vi "Laser Rough Cutting.vi"(0 "configuration file path":path caption="配置文件的路径", 1 "rough cutting msic":T1) -> ()   [LabVIEW 2014]
uses:
  Ctl.xio/rough cutting msic ctl.ctl
  SubVIS.xio/DataSocket/DataSocket_Tags.ctl
  Ctl.xio/part type.ctl
  SubVIS.xio/Creat Write List VI's/DefCtrl/Station.ctl
  SubVIS.xio/DataSocket/Write PLC Vars/Write String Var in.vi
  <vilib>/Utility/file.llb/Read From Spreadsheet File (string).vi
  SubVIS.xio/DataSocket/Write PLC Vars/Write Bool Var in.vi
  SubVIS.xio/DataSocket/Read PLC Vars/Read String Var.vi
  SubVIS.xio/DataSocket/Write PLC Vars/Write Dbl Var in.vi
  SubVIS.xio/DataSocket/Read PLC Vars/Read Bool Var.vi
  SubVIS.xio/DataSocket/Read PLC Vars/Read U32 Var.vi
panel:
  in  "SQL information":string
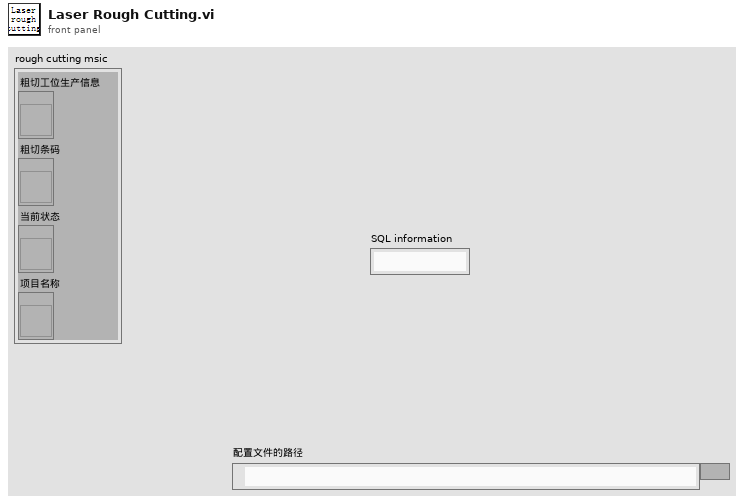
[diagram p1: front panel]
types:
  T1 = cluster{"粗切工位生产信息":refnum<vi>, "粗切条码":refnum<vi>, "当前状态":refnum<vi>, "项目名称":refnum<vi>}
  T2 = typedef "Station.ctl" = enum16{"粗切工位", "热处理工位", "精切工位", "PDF焊接工位", "打凹点预载力工位", "收卷工位", "EOL工位"}
  T3 = typedef "rough cutting msic ctl.ctl" = cluster{"configuration file path":path, "DsOut":T4[], "scanner coms or ip":string, "BarCode":string, "scanner resource name out":refnum<visa-resource-name>, "Hopper car information":cluster{"Hopper car code":string, "Hopper car No":string, "plate No":string}, "pallet.produced number":i32, "SQL information":string, "Database":string[], "Serial number":i32, "database path":path, "rough cutting msic":cluster{"粗切工位生产信息":refnum<vi>, "粗切条码":refnum<vi>, "当前状态":refnum<vi>, "项目名称":refnum<vi>}, "part type":T5, "scanner ip ID":refnum<k5>, "Number of scans ":u8}
  T4 = typedef "DataSocket_Tags.ctl" = cluster{"Ds ID":refnum<k13>, "Tag":string}
  T5 = typedef "part type.ctl" = cluster{"项目号":string, "物料代码":string, "零件号":string, "供应商编码":string, "产线编码":string, "客户代码":string, "颜色代码":string, "托盘上限":i32, "加热温度":string, "加热时长":string, "EOL Stations":string}
  T6 = cluster{"Hopper car code":string, "Hopper car No":string, "plate No":string}
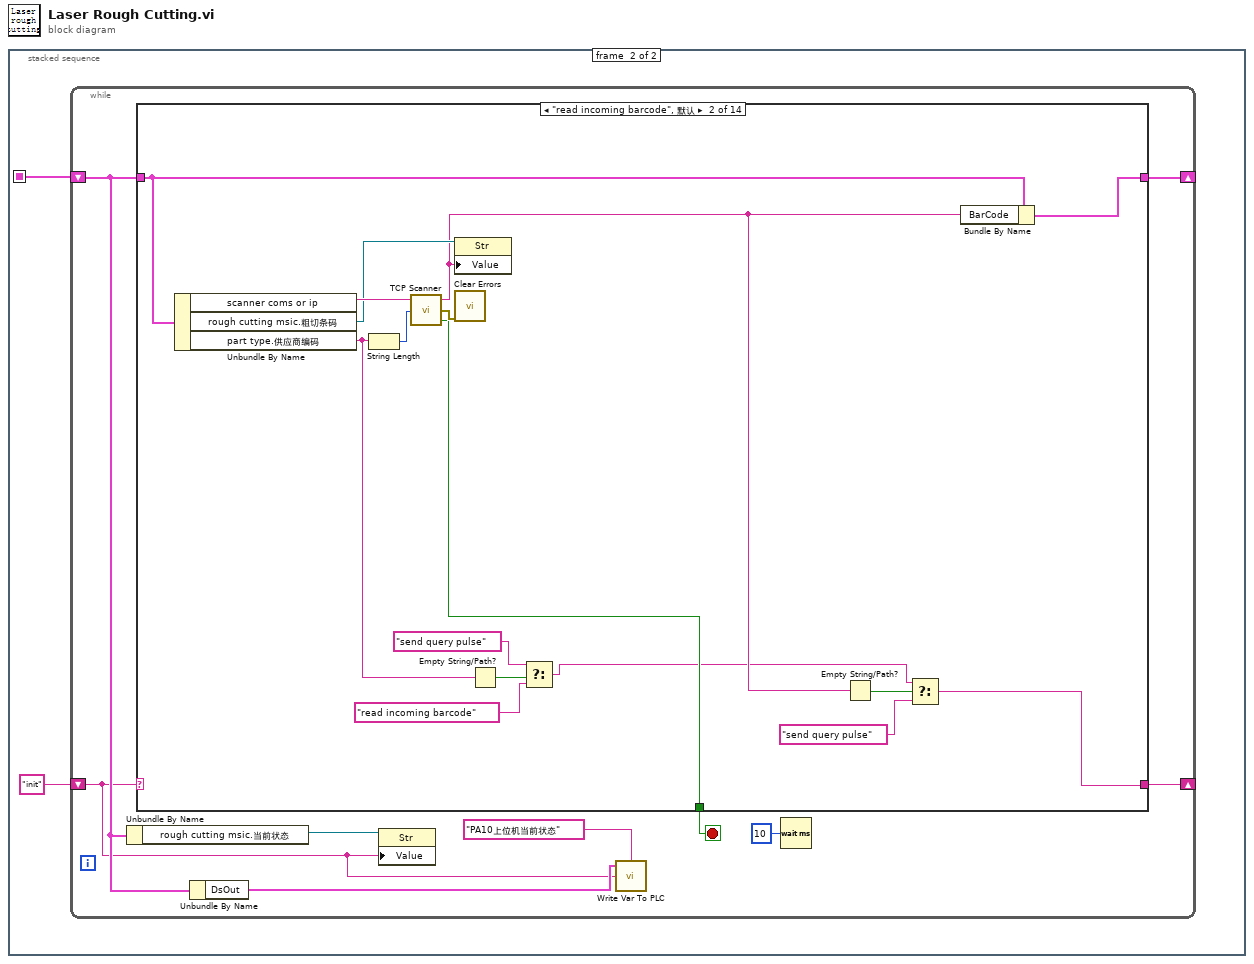
[diagram p0: block diagram]
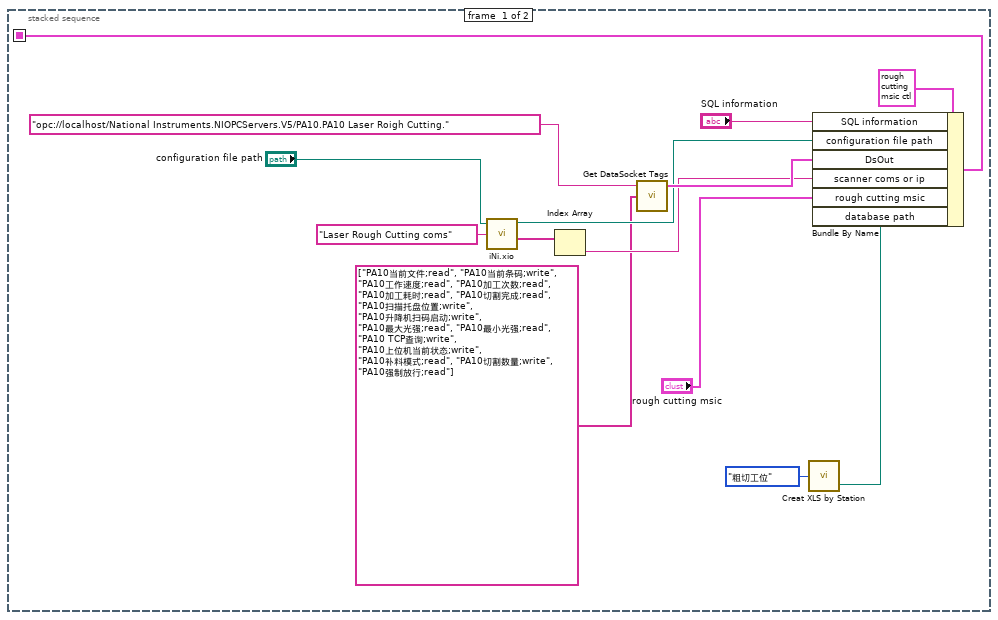
[diagram p2: hidden frame]
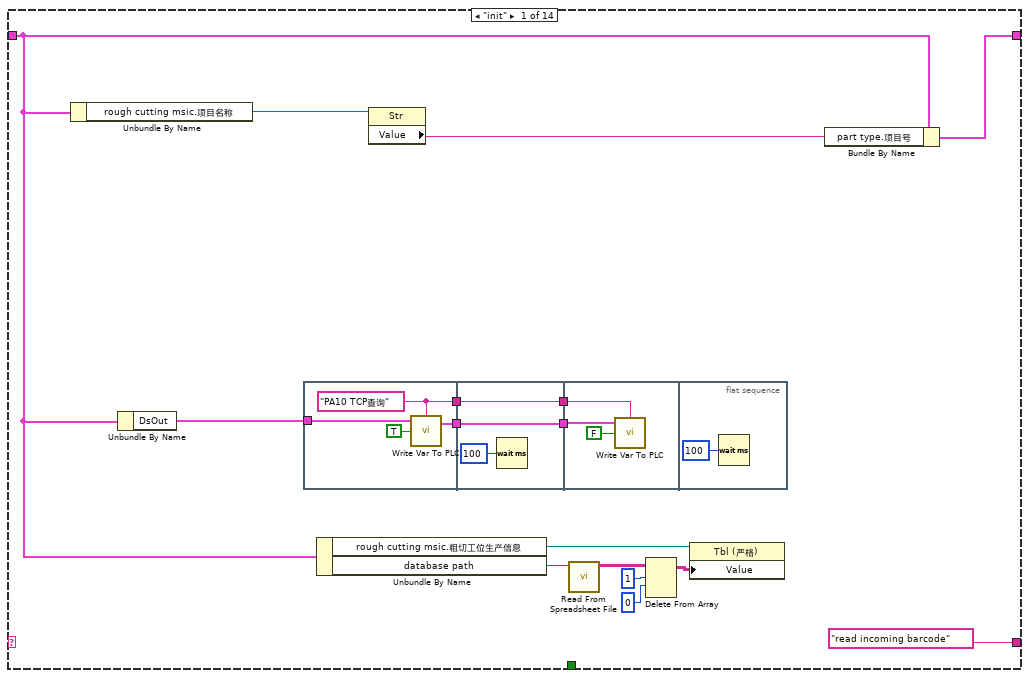
[diagram p3: hidden frame]
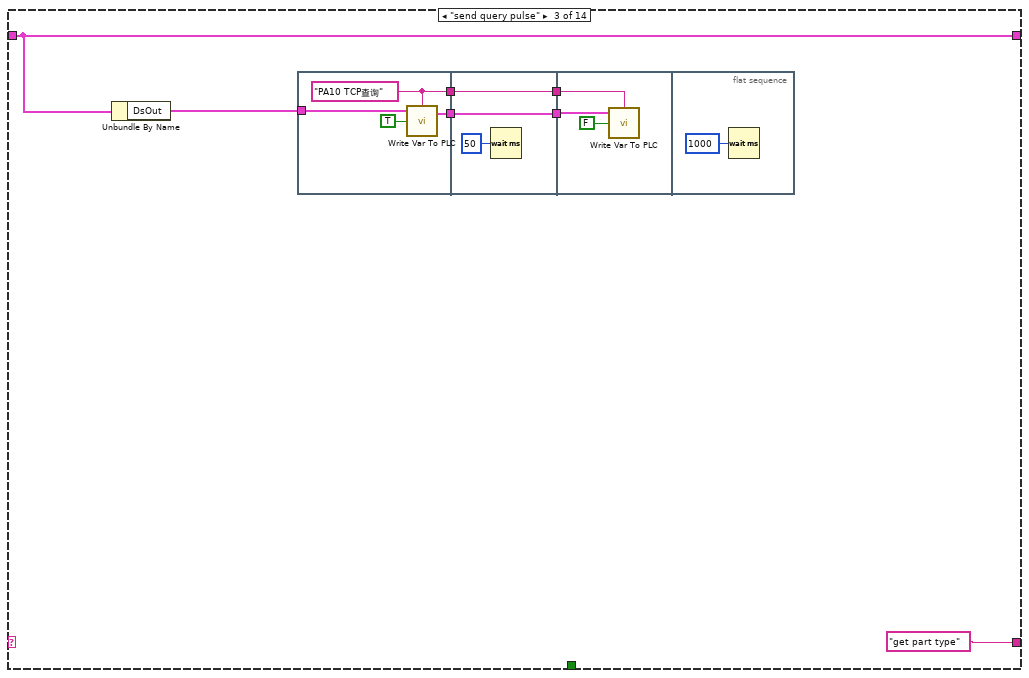
[diagram p4: hidden frame]
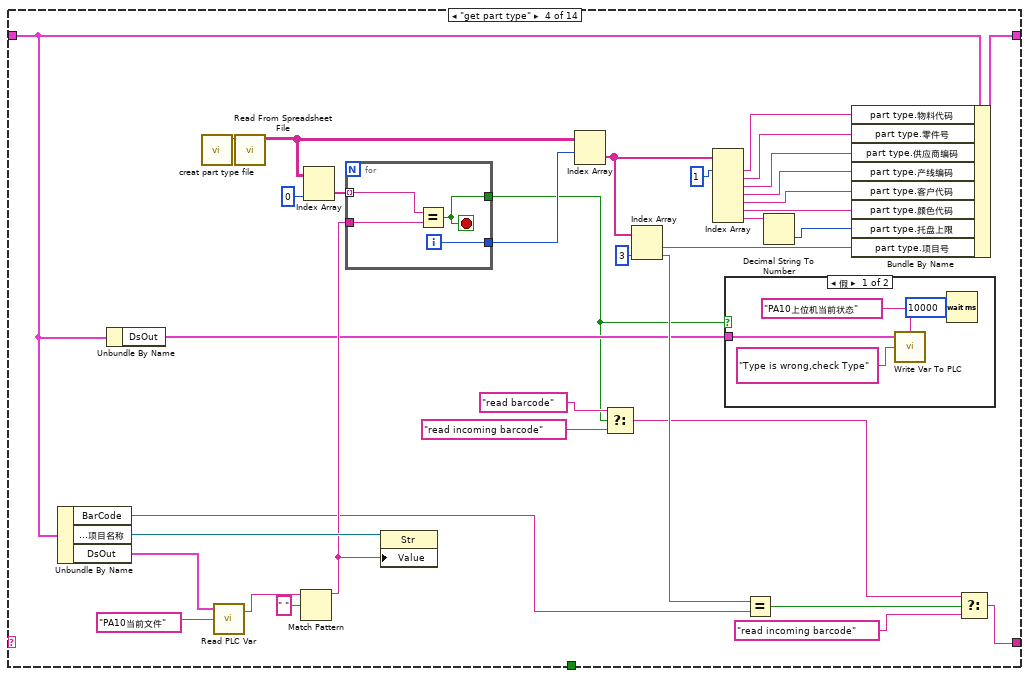
[diagram p5: hidden frame]
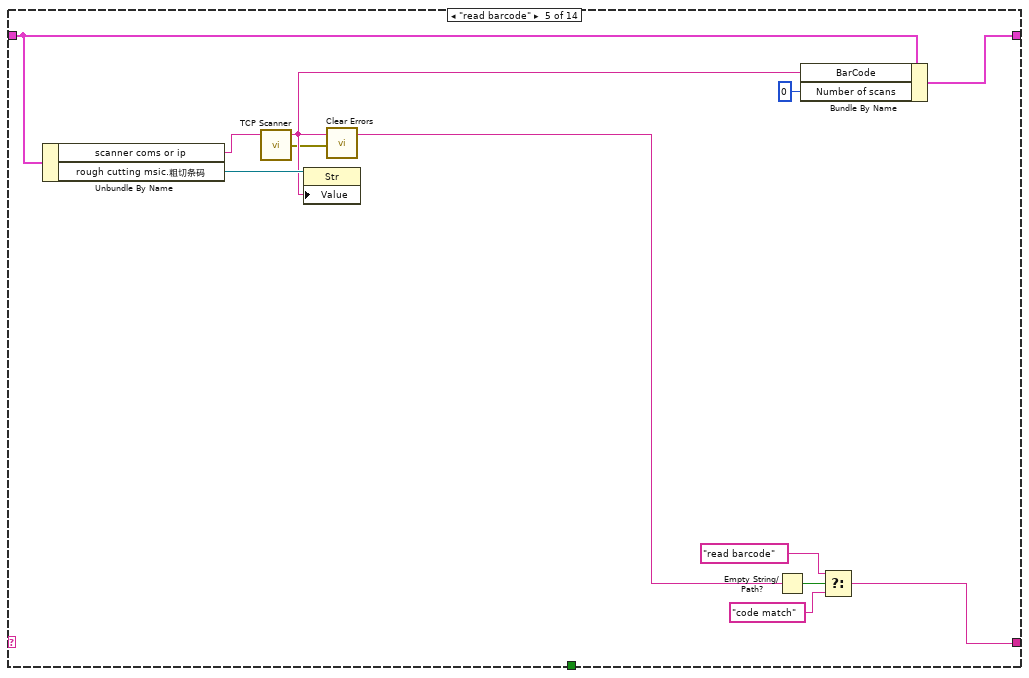
[diagram p7: hidden frame]
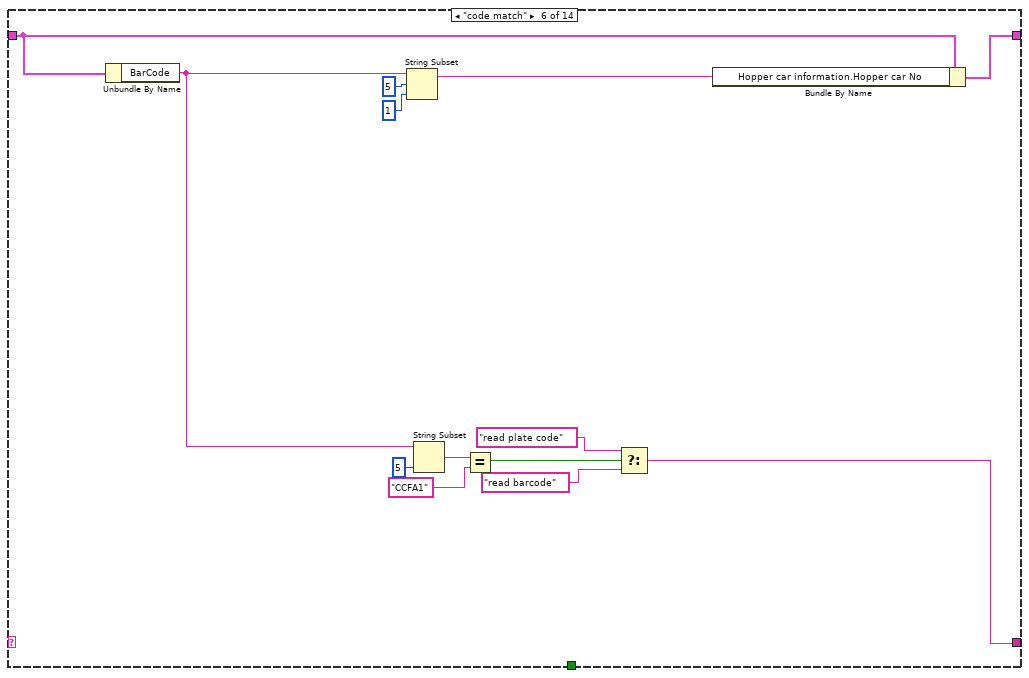
[diagram p8: hidden frame]
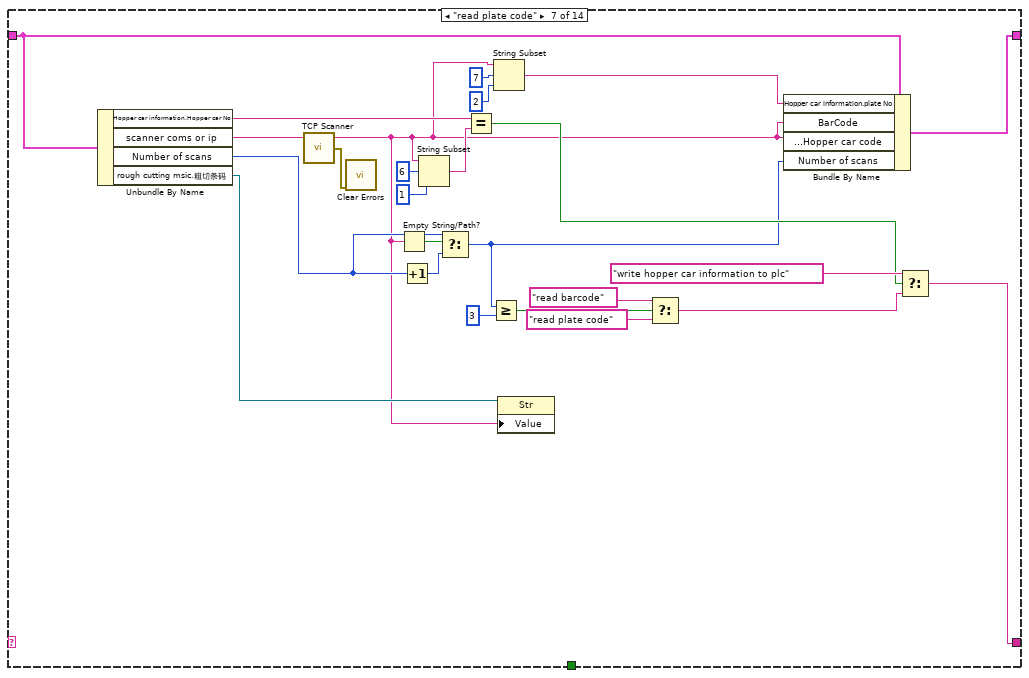
[diagram p9: hidden frame]
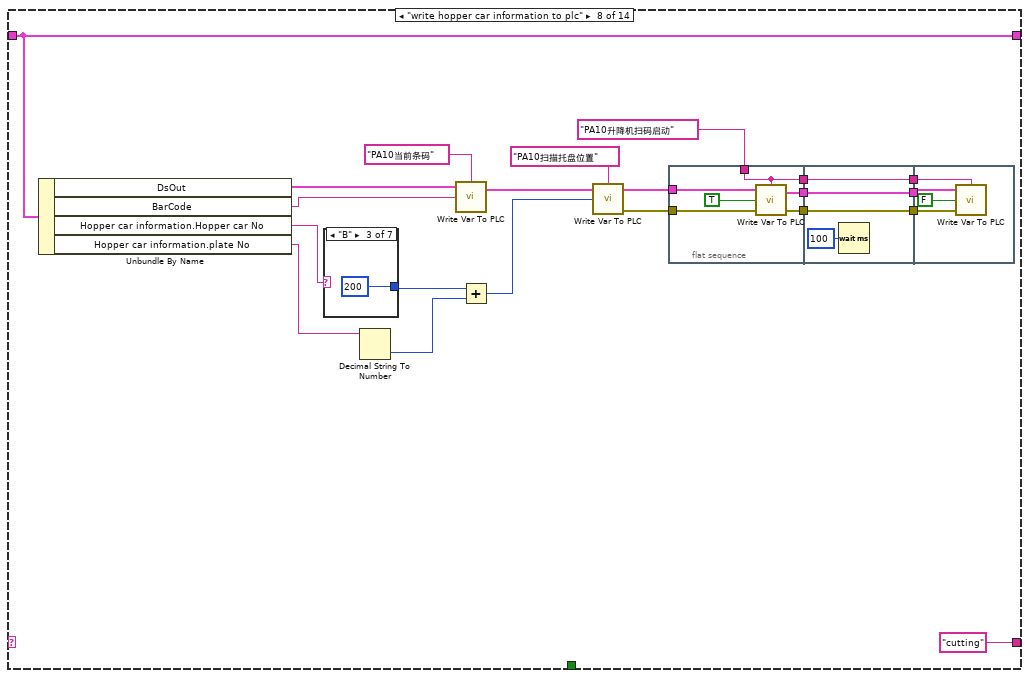
[diagram p10: hidden frame]
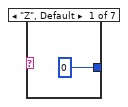
[diagram p11: hidden frame]
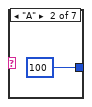
[diagram p12: hidden frame]
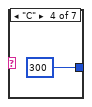
[diagram p13: hidden frame]
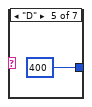
[diagram p14: hidden frame]
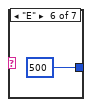
[diagram p15: hidden frame]
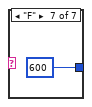
[diagram p16: hidden frame]
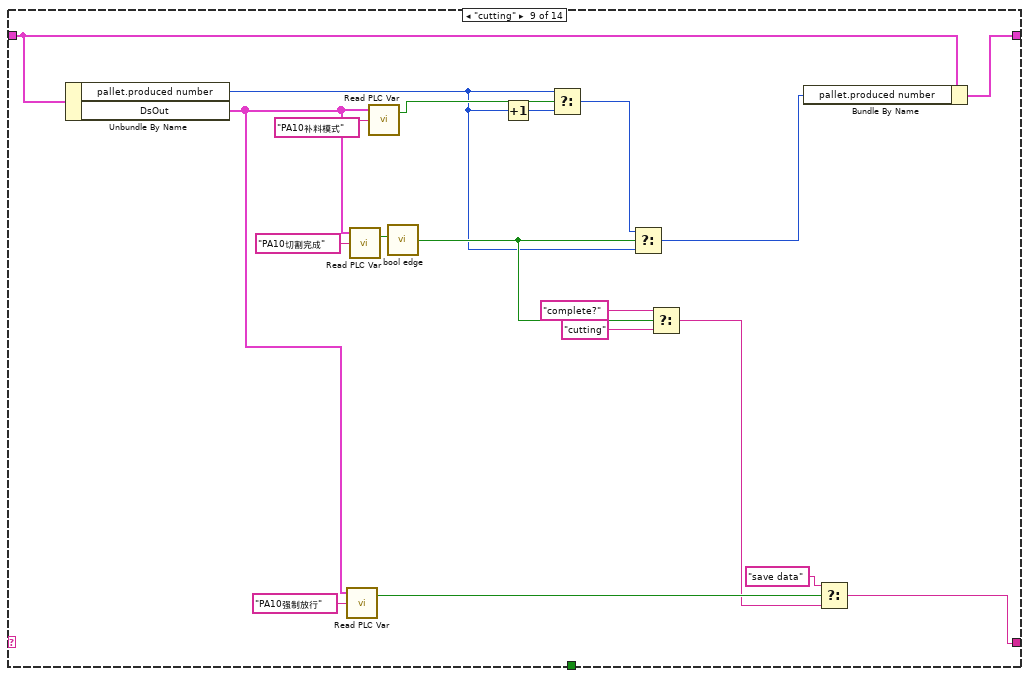
[diagram p17: hidden frame]
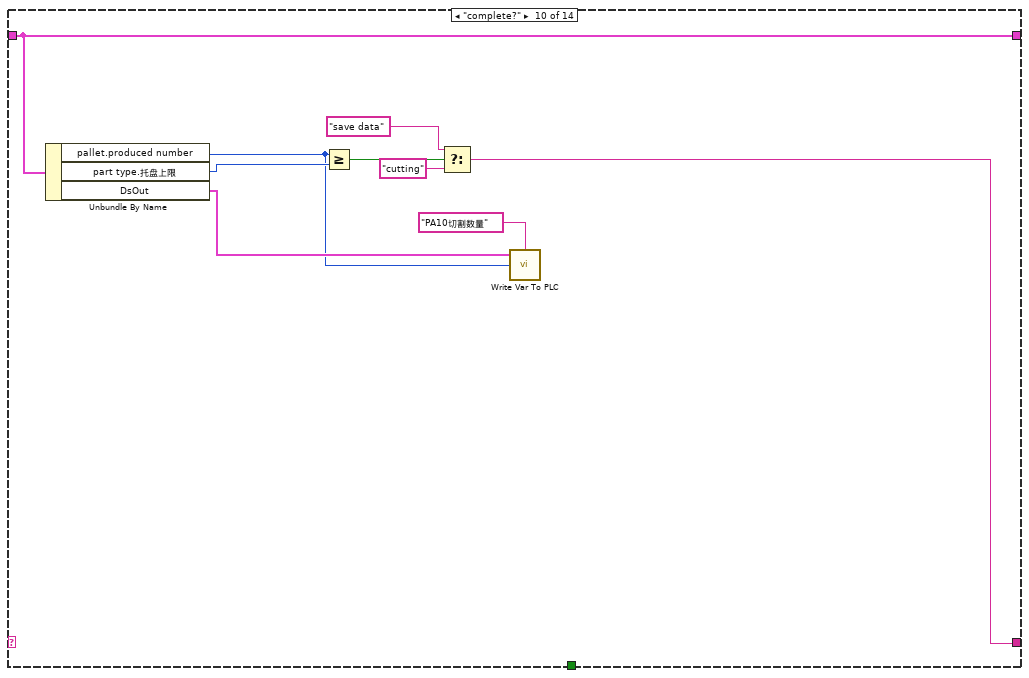
[diagram p18: hidden frame]
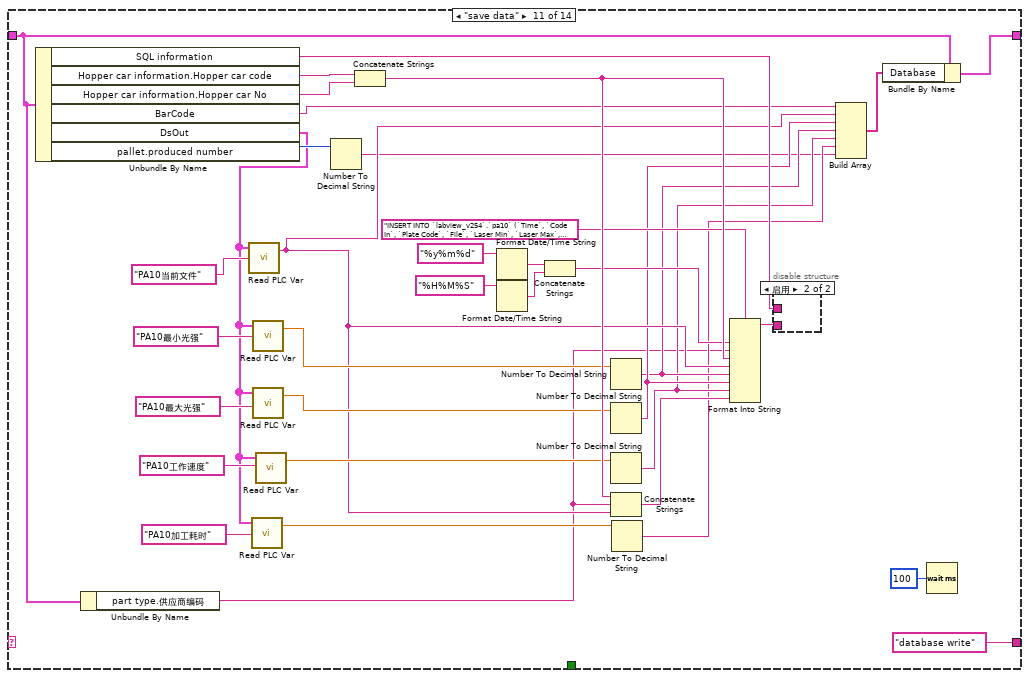
[diagram p19: hidden frame]
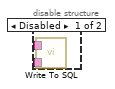
[diagram p20: hidden frame]
diagram:
  n1 = stacked-sequence {
    seq-local: [w3 _] -> [_ w15]
    frame #0 {
      n2 = call "iNi.xio.vi"("configuration file path"="configuration file path", "Sections"="Laser Rough Cutting coms") -> ("configuration file path"=w13:path, "Values"=w11:string[])  [unwired: 1 in, 3 out]
      n3 = Index Array(array=w11) -> (element=w10:string)  [unwired: 1 in]
      n4 = call "Get DataSocket Tags.vi"("All Tags"=string[] ["PA10当前文件;read", "PA10当前条码;write", "PA10工作速度;read", "PA10加工次数;read", "PA10加工耗时;read", "PA10切割完成;read", "PA10扫描托盘位置;write", "PA10升降机扫码启动;write", "PA10最大光强;read", "PA10最小光强;read", "PA10 TCP查询;write", "PA10上位机当前状态;write", "PA10补料模式;read", "PA10切割数量;write", "PA10强制放行;read"], "URL"="opc://localhost/National Instruments.NIOPCServers.V5/PA10.PA10 Laser Roigh Cutting.") -> ("DsOut"=w14:T4[])  [unwired: 3 in]
      n5 = call "Creat XLS by Station.vi"("staiton"=Station."粗切工位") -> ("new file path (Not A Path if cancelled)"=w2:path)  [unwired: 5 in]
      n6 = Bundle By Name(cluster=T3 {"configuration file path"=path "", "DsOut"=[], "scanner coms or ip"="", "BarCode"="", "scanner resource name out"="", "Hopper car information"={"Hopper car code"="", "Hopper car No"="", "plate No"=""}, "pallet.produced number"=0, "SQL information"="", "Database"=[], "Serial number"=0, "database path"=path "", "rough cutting msic"={"粗切工位生产信息"=refnum, "粗切条码"=refnum, "当前状态"=refnum, "项目名称"=refnum}, "part type"={"项目号"="", "物料代码"="", "零件号"="", "供应商编码"="", "产线编码"="", "客户代码"="", "颜色代码"="", "托盘上限"=0, "加热温度"="", "加热时长"="", "EOL Stations"=""}, "scanner ip ID"=refnum, "Number of scans "=0} ("rough cutting msic"), "SQL information"="SQL information", "configuration file path"=w13, "DsOut"=w14, "scanner coms or ip"=w10, "rough cutting msic"="rough cutting msic", "database path"=w2) -> (w3:T3)
    }
    frame #1 {
      n7 = while {
        shift-right: [w25] -> _
        shift-left: w15 -> [w20]
        shift-right: [w24] -> _
        shift-left: "init" ("event") -> [w18]
        stop <- w17 stop-if-true
        n8 = Unbundle By Name(w20) -> ("rough cutting msic.当前状态"=w22:refnum<vi>)
        n9 = case shown="\"read incoming barcode\", 默认" w18 {
          tunnel: w20 -> [w26 w65 w70 w89 w138 w142 w171 w179 w237 w243 w251 w300 w314 w321]
          tunnel: [w41 w68 w70 w121 w137 w150 w170 w179 w239 w243 w256 w307 w314 w326] -> w25
          tunnel: ["read incoming barcode" w59 "get part type" ("f") w114 w133 w148 w173 "cutting" ("event") w222 w246 "database write" ("f") "updata display" ("f") "reset" ("f") "read incoming barcode" ("f")] -> w24
          tunnel: [_ w58 _ _ _ _ _ _ _ _ _ _ _ _] -> w17
          frame "init" {
            n10 = Unbundle By Name(w26) -> ("rough cutting msic.项目名称"=w39:refnum<vi>)
            n11 = Unbundle By Name(w26) -> ("DsOut"=w33:T4[])
            n12 = flat-sequence {
              tunnel: w33 -> [w45]
              tunnel: [w43] -> w37
              tunnel: [w42] -> w36
              tunnel: w37 -> [w47]
              tunnel: [w47] -> w35
              tunnel: w36 -> [w46]
              tunnel: [w46] -> w34
              tunnel: w35 -> [w51]
              tunnel: w34 -> [w49]
              frame #0 {
                w42 = "PA10 TCP查询" ("Tag IN")
                n13 = call-poly "Write Var To PLC.vi"("Tag IN"=w42, "Bool Var in"=TRUE, "Ds PLCTags IN"=w45) -> ("Ds PLCTags OUT"=w43:T4[])  [unwired: 1 in, 1 out]
              }
              frame #1 {
                n14 = Wait (ms)(milliseconds to wait=u32 100 ("等待时间（毫秒）")) -> ()  [unwired: 1 out]
              }
              frame #2 {
                n15 = call-poly "Write Var To PLC.vi"("Tag IN"=w49, "Bool Var in"=FALSE, "Ds PLCTags IN"=w51) -> ()  [unwired: 1 in, 2 out]
              }
              frame #3 {
                n16 = Wait (ms)(milliseconds to wait=u32 100 ("等待时间（毫秒）")) -> ()  [unwired: 1 out]
              }
            }
            n17 = Unbundle By Name(w26) -> ("rough cutting msic.粗切工位生产信息"=w32:refnum<vi>, "database path"=w31:path)
            n18 = property class="Str"(reference=w39) -> ("Value"=w38:string)  [unwired: 1 in, 2 out]
            n19 = call-poly <vilib>:"Read From Spreadsheet File.vi"("file path (dialog if empty)"=w31) -> ("all rows"=w30:string[][])  [unwired: 6 in, 4 out]
            n20 = Delete From Array(array=w30, length=1 ("长度"), index (row)=0 ("索引 (行)")) -> (array with subset deleted=w27:string[][])  [unwired: 1 in, 1 out]
            n21 = property class="Tbl (严格)"(reference=w32, "Value"=w27) -> ()  [unwired: 1 in, 2 out]
            n22 = Bundle By Name(cluster=w26, "part type.项目号"=w38) -> (w41:T3)
          }
          frame "read incoming barcode", Default {
            n23 = Unbundle By Name(w65) -> ("scanner coms or ip"=w67:string, "rough cutting msic.粗切条码"=w66:refnum<vi>, "part type.供应商编码"=w56:string)
            n24 = String Length(string=w56) -> (length=w64:i32)
            n25 = call "TCP Scanner.vi"("byte of read(9)"=w64, "ip"=w67) -> ("status"=w58:bool, "错误输出"=w63:errorcluster, "Barcode"=w62:string)  [unwired: 1 in]
            n26 = property class="Str"(reference=w66, "Value"=w62) -> ()  [unwired: 1 in, 2 out]
            n27 = call <vilib>:"Clear Errors.vi"("error in (no error)"=w63) -> ()  [unwired: 5 in, 2 out]
            n28 = Empty String/Path?(string/path=w56) -> (empty?=w57:bool)
            n29 = Select(t="send query pulse" ("f"), s=w57, f="read incoming barcode") -> (s? t:f=w53:string)
            n30 = Empty String/Path?(string/path=w62) -> (empty?=w61:bool)
            n31 = Select(t=w53, s=w61, f="send query pulse") -> (s? t:f=w59:string)
            n32 = Bundle By Name(cluster=w65, "BarCode"=w62) -> (w68:T3)
          }
          frame "send query pulse" {
            n33 = Unbundle By Name(w70) -> ("DsOut"=w71:T4[])
            n34 = flat-sequence {
              tunnel: w71 -> [w79]
              tunnel: [w77] -> w75
              tunnel: [w76] -> w74
              tunnel: w75 -> [w81]
              tunnel: [w81] -> w73
              tunnel: w74 -> [w80]
              tunnel: [w80] -> w72
              tunnel: w73 -> [w85]
              tunnel: w72 -> [w83]
              frame #0 {
                w76 = "PA10 TCP查询" ("Tag IN")
                n35 = call-poly "Write Var To PLC.vi"("Tag IN"=w76, "Bool Var in"=TRUE, "Ds PLCTags IN"=w79) -> ("Ds PLCTags OUT"=w77:T4[])  [unwired: 1 in, 1 out]
              }
              frame #1 {
                n36 = Wait (ms)(milliseconds to wait=u32 50 ("等待时间（毫秒）")) -> ()  [unwired: 1 out]
              }
              frame #2 {
                n37 = call-poly "Write Var To PLC.vi"("Tag IN"=w83, "Bool Var in"=FALSE, "Ds PLCTags IN"=w85) -> ()  [unwired: 1 in, 2 out]
              }
              frame #3 {
                n38 = Wait (ms)(milliseconds to wait=u32 1000 ("等待时间（毫秒）")) -> ()  [unwired: 1 out]
              }
            }
          }
          frame "get part type" {
            n39 = Unbundle By Name(w89) -> ("BarCode"=w95:string, "rough cutting msic.项目名称"=w97:refnum<vi>, "DsOut"=w104:T4[])
            n40 = Unbundle By Name(w89) -> ("DsOut"=w88:T4[])
            n41 = call "creat part type file.vi"() -> ("new file path (Not A Path if cancelled)"=w115:path)  [unwired: 11 in]
            n42 = call-poly "Read PLC Var.vi"("Tag IN"="PA10当前文件", "Ds PLCTags IN"=w104) -> ("String Var out"=w99:string)  [unwired: 1 in, 1 out]
            n43 = call-poly <vilib>:"Read From Spreadsheet File.vi"("file path (dialog if empty)"=w115) -> ("all rows"=w117:string[][])  [unwired: 6 in, 4 out]
            n44 = Match Pattern(string=w99, regular expression=" " ("正则表达式")) -> (before substring=w96:string)  [unwired: 1 in, 3 out]
            n45 = Index Array(array=w117, index (col)=0 ("禁用的索引 (列)")) -> (element=w118:string[])  [unwired: 1 in]
            n46 = for {
              tunnel: w118 -> [w127] mode=indexing
              tunnel: [w129] -> w116
              tunnel: w96 -> [w128]
              tunnel: [w126] -> w87
              i -> [w129]
              stop <- w126 stop-if-true
              n47 = Equal?(x=w127, y=w128) -> (x = y?=w126:bool)
            }
            n48 = property class="Str"(reference=w97, "Value"=w96) -> ()  [unwired: 1 in, 2 out]
            n49 = Index Array(array=w117, index (row)=w116) -> (element=w103:string[])  [unwired: 1 in]
            n50 = Select(t="read barcode", s=w87, f="read incoming barcode") -> (s? t:f=w90:string)
            n51 = Index Array(array=w103, index #2=3 ("索引")) -> (element #1=w101:string, element #2=w94:string)  [unwired: 1 in]
            n52 = Index Array(array=w103, index #1=1 ("索引")) -> (element #1=w112:string, element #2=w111:string, element #3=w110:string, element #4=w109:string, element #5=w108:string, element #6=w107:string, element #7=w106:string)  [unwired: 6 in]
            n53 = case shown="假" w87 {
              tunnel: w88 -> [w125 _]
              frame False {
                n54 = call-poly "Write Var To PLC.vi"("Tag IN"="PA10上位机当前状态", "String Var in"="Type is wrong,check Type", "Ds PLCTags IN"=w125) -> ()  [unwired: 1 in, 2 out]
                n55 = Wait (ms)(milliseconds to wait=u32 10000 ("等待时间（毫秒）")) -> ()  [unwired: 1 out]
              }
              frame True {
              }
            }
            n56 = Equal?(x=w94, y=w95) -> (x = y?=w102:bool)
            n57 = Decimal String To Number(string=w106) -> (number=w113:i32)  [unwired: 2 in, 1 out]
            n58 = Bundle By Name(cluster=w89, "part type.物料代码"=w112, "part type.零件号"=w111, "part type.供应商编码"=w110, "part type.产线编码"=w109, "part type.客户代码"=w108, "part type.颜色代码"=w107, "part type.托盘上限"=w113, "part type.项目号"=w101) -> (w121:T3)
            n59 = Select(t=w90, s=w102, f="read incoming barcode") -> (s? t:f=w114:string)
          }
          frame "read barcode" {
            n60 = Unbundle By Name(w138) -> ("scanner coms or ip"=w140:string, "rough cutting msic.粗切条码"=w139:refnum<vi>)
            n61 = call "TCP Scanner.vi"("ip"=w140) -> ("错误输出"=w131:errorcluster, "Barcode"=w132:string)  [unwired: 2 in, 1 out]
            n62 = property class="Str"(reference=w139, "Value"=w132) -> ()  [unwired: 1 in, 2 out]
            n63 = call <vilib>:"Clear Errors.vi"("error in (no error)"=w131) -> ()  [unwired: 5 in, 2 out]
            n64 = Empty String/Path?(string/path=w132) -> (empty?=w136:bool)
            n65 = Bundle By Name(cluster=w138, "BarCode"=w132, "Number of scans"=u8 0) -> (w137:T3)
            n66 = Select(t="read barcode", s=w136, f="code match") -> (s? t:f=w133:string)
          }
          frame "code match" {
            n67 = Unbundle By Name(w142) -> ("BarCode"=w141:string)
            n68 = String Subset(string=w141, offset (0)=5 ("偏移量(0)"), length (rest)=1 ("长度（剩余）")) -> (substring=w144:string)
            n69 = String Subset(string=w141, length (rest)=5 ("长度（剩余）")) -> (substring=w145:string)  [unwired: 1 in]
            n70 = Equal?(x=w145, y="CCFA1") -> (x = y?=w149:bool)
            n71 = Select(t="read plate code" ("event"), s=w149, f="read barcode" ("event")) -> (s? t:f=w148:string)
            n72 = Bundle By Name(cluster=w142, "Hopper car information.Hopper car No"=w144) -> (w150:T3)
          }
          frame "read plate code" {
            n73 = Unbundle By Name(w171) -> ("Hopper car information.Hopper car No"=w175:string, "scanner coms or ip"=w178:string, "Number of scans"=w161:u8, "rough cutting msic.粗切条码"=w158:refnum<vi>)
            n74 = call "TCP Scanner.vi"("ip"=w178) -> ("错误输出"=w163:errorcluster, "Barcode"=w155:string)  [unwired: 2 in, 1 out]
            n75 = call <vilib>:"Clear Errors.vi"("error in (no error)"=w163) -> ()  [unwired: 5 in, 2 out]
            n76 = Empty String/Path?(string/path=w155) -> (empty?=w162:bool)
            n77 = Increment(x=w161) -> (x+1=w160:u8)
            n78 = String Subset(string=w155, offset (0)=6 ("偏移量(0)"), length (rest)=1 ("长度（剩余）")) -> (substring=w169:string)
            n79 = Select(t=w161, s=w162, f=w160) -> (s? t:f=w159:u8)
            n80 = Equal?(x=w175, y=w169) -> (x = y?=w172:bool)
            n81 = Greater Or Equal?(x=w159, y=u8 3) -> (x >= y?=w167:bool)
            n82 = String Subset(string=w155, offset (0)=7 ("偏移量(0)"), length (rest)=2 ("长度（剩余）")) -> (substring=w154:string)
            n83 = property class="Str"(reference=w158, "Value"=w155) -> ()  [unwired: 1 in, 2 out]
            n84 = Select(t="read barcode" ("event"), s=w167, f="read plate code" ("event")) -> (s? t:f=w164:string)
            n85 = Bundle By Name(cluster=w171, "Hopper car information.plate No"=w154, "BarCode"=w155, "Hopper car information.Hopper car code"=w155, "Number of scans"=w159) -> (w170:T3)
            n86 = Select(t="write hopper car information to plc" ("event"), s=w172, f=w164) -> (s? t:f=w173:string)
          }
          frame "write hopper car information to plc" {
            n87 = Unbundle By Name(w179) -> ("DsOut"=w182:T4[], "BarCode"=w181:string, "Hopper car information.Hopper car No"=w199:string, "Hopper car information.plate No"=w198:string)
            n88 = case shown="\"B\"" w199 {
              tunnel: [0 100 200 300 400 500 600] -> w197
              frame "Z", Default {
              }
              frame "A" {
              }
              frame "B" {
              }
              frame "C" {
              }
              frame "D" {
              }
              frame "E" {
              }
              frame "F" {
              }
            }
            n89 = Decimal String To Number(string=w198) -> (number=w196:i32)  [unwired: 2 in, 1 out]
            n90 = call-poly "Write Var To PLC.vi"("Tag IN"="PA10当前条码", "String Var in"=w181, "Ds PLCTags IN"=w182) -> ("Ds PLCTags OUT"=w183:T4[])  [unwired: 1 in, 1 out]
            n91 = Add(x=w197, y=w196) -> (x+y=w194:i32)
            n92 = call-poly "Write Var To PLC.vi"("Tag IN"="PA10扫描托盘位置", "Dbl Var in"=w194, "Ds PLCTags IN"=w183) -> ("error out"=w193:errorcluster, "Ds PLCTags OUT"=w192:T4[])  [unwired: 1 in]
            n93 = flat-sequence {
              tunnel: w193 -> [w205]
              tunnel: w192 -> [w204]
              tunnel: "PA10升降机扫码启动" ("Tag IN") -> [w201]
              tunnel: [w202] -> w188
              tunnel: [w201] -> w187
              tunnel: [w200] -> w185
              tunnel: [w208] -> w189
              tunnel: w188 -> [w208]
              tunnel: w187 -> [w207]
              tunnel: [w207] -> w186
              tunnel: w185 -> [w206]
              tunnel: [w206] -> w184
              tunnel: w189 -> [w213]
              tunnel: w186 -> [w212]
              tunnel: w184 -> [w211]
              frame #0 {
                n94 = call-poly "Write Var To PLC.vi"("Tag IN"=w201, "错误输入（无错误）"=w205, "Bool Var in"=TRUE, "Ds PLCTags IN"=w204) -> ("error out"=w200:errorcluster, "Ds PLCTags OUT"=w202:T4[])
              }
              frame #1 {
                n95 = Wait (ms)(milliseconds to wait=u32 100 ("等待时间（毫秒）")) -> ()  [unwired: 1 out]
              }
              frame #2 {
                n96 = call-poly "Write Var To PLC.vi"("Tag IN"=w212, "错误输入（无错误）"=w211, "Bool Var in"=FALSE, "Ds PLCTags IN"=w213) -> ()  [unwired: 2 out]
              }
            }
          }
          frame "cutting" {
            n97 = Unbundle By Name(w237) -> ("pallet.produced number"=w228:i32, "DsOut"=w225:T4[])
            n98 = call-poly "Read PLC Var.vi"("Tag IN"="PA10强制放行", "Ds PLCTags IN"=w225) -> ("Bool Var out"=w224:bool)  [unwired: 1 in, 1 out]
            n99 = call-poly "Read PLC Var.vi"("Tag IN"="PA10切割完成", "Ds PLCTags IN"=w225) -> ("Bool Var out"=w232:bool)  [unwired: 1 in, 1 out]
            n100 = call-poly "Read PLC Var.vi"("Tag IN"="PA10补料模式", "Ds PLCTags IN"=w225) -> ("Bool Var out"=w230:bool)  [unwired: 1 in, 1 out]
            n101 = call "bool edge.vi"("bool in"=w232) -> ("true-false"=w236:bool)  [unwired: 6 in, 1 out]
            n102 = Increment(x=w228) -> (x+1=w229:i32)
            n103 = Select(t=w228, s=w230, f=w229) -> (s? t:f=w227:i32)
            n104 = Select(t=w227, s=w236, f=w228) -> (s? t:f=w238:i32)
            n105 = Select(t="complete?" ("event"), s=w236, f="cutting" ("event")) -> (s? t:f=w223:string)
            n106 = Bundle By Name(cluster=w237, "pallet.produced number"=w238) -> (w239:T3)
            n107 = Select(t="save data" ("event"), s=w224, f=w223) -> (s? t:f=w222:string)
          }
          frame "complete?" {
            n108 = Unbundle By Name(w243) -> ("pallet.produced number"=w241:i32, "part type.托盘上限"=w248:i32, "DsOut"=w242:T4[])
            n109 = Greater Or Equal?(x=w241, y=w248) -> (x >= y?=w247:bool)
            n110 = Select(t="save data" ("event"), s=w247, f="cutting") -> (s? t:f=w246:string)
            n111 = call-poly "Write Var To PLC.vi"("Tag IN"="PA10切割数量", "Dbl Var in"=w241, "Ds PLCTags IN"=w242) -> ()  [unwired: 1 in, 2 out]
          }
          frame "save data" {
            n112 = Unbundle By Name(w251) -> ("SQL information"=w266:string, "Hopper car information.Hopper car code"=w268:string, "Hopper car information.Hopper car No"=w267:string, "BarCode"=w253:string, "DsOut"=w252:T4[], "pallet.produced number"=w255:i32)
            n113 = Unbundle By Name(w251) -> ("part type.供应商编码"=w250:string)
            n114 = call-poly "Read PLC Var.vi"("Tag IN"="PA10当前文件", "Ds PLCTags IN"=w252) -> ("String Var out"=w264:string)  [unwired: 1 in, 1 out]
            n115 = call-poly "Read PLC Var.vi"("Tag IN"="PA10加工耗时", "Ds PLCTags IN"=w252) -> ("U32 Var out"=w259:dbl)  [unwired: 1 in, 1 out]
            n116 = call-poly "Read PLC Var.vi"("Tag IN"="PA10最小光强", "Ds PLCTags IN"=w252) -> ("U32 Var out"=w273:dbl)  [unwired: 1 in, 1 out]
            n117 = call-poly "Read PLC Var.vi"("Tag IN"="PA10最大光强", "Ds PLCTags IN"=w252) -> ("U32 Var out"=w271:dbl)  [unwired: 1 in, 1 out]
            n118 = call-poly "Read PLC Var.vi"("Tag IN"="PA10工作速度", "Ds PLCTags IN"=w252) -> ("U32 Var out"=w269:dbl)  [unwired: 1 in, 1 out]
            n119 = Number To Decimal String(number=w255) -> (decimal integer string=w254:string)  [unwired: 1 in]
            n120 = Concatenate Strings(w268, w267) -> (w284:string)
            n121 = Format Date/Time String(time format string (%c)="%y%m%d" ("时间格式字符串(%c)")) -> (date/time string=w279:string)  [unwired: 2 in]
            n122 = Format Date/Time String(time format string (%c)="%H%M%S" ("时间格式字符串(%c)")) -> (date/time string=w278:string)  [unwired: 2 in]
            n123 = Concatenate Strings(w279, w278) -> (w276:string)
            n124 = Number To Decimal String(number=w273) -> (decimal integer string=w262:string)  [unwired: 1 in]
            n125 = Number To Decimal String(number=w271) -> (decimal integer string=w263:string)  [unwired: 1 in]
            n126 = Number To Decimal String(number=w269) -> (decimal integer string=w261:string)  [unwired: 1 in]
            n127 = Concatenate Strings(w284, w250, w264) -> (w281:string)
            n128 = Number To Decimal String(number=w259) -> (decimal integer string=w258:string)  [unwired: 1 in]
            n129 = Format Into String(format string="INSERT INTO `labview_v254`.`pa10` (`Time`, `Code In`, `Plate Code`, `File`, `Laser Min`, `Laser Max`, `Vel`, `Code Out`) VALUES ('%s', '%s', '%s', '%s', '%s', '%s', '%s', '%s');", w276, w250, w284, w264, w262, w263, w261, w281) -> (resulting string=w282:string)  [unwired: 2 in, 1 out]
            n130 = disable-structure shown="启用" {
              disable-tunnel: w282 -> [w286 _]
              disable-tunnel: w266 -> [w285 _]
              frame Disabled {
                n131 = call "Write To SQL.vi"("SQL query"=w286, "connection information"=w285) -> ()  [unwired: 1 out]
              }
              frame Enabled {
              }
            }
            n132 = Build Array(w253, w264, w263, w262, w261, w258, w254) -> (w257:string[])
            n133 = Bundle By Name(cluster=w251, "Database"=w257) -> (w256:T3)
            n134 = Wait (ms)(milliseconds to wait=u32 100 ("等待时间（毫秒）")) -> ()  [unwired: 1 out]
          }
          frame "database write" {
            w297 = enum16{"read", "write"}."write" ("write\\read")
            n135 = Unbundle By Name(w300) -> ("configuration file path"=w299:path, "BarCode"=w296:string)
            n136 = Unbundle By Name(w300) -> ("Database"=w306:string[], "part type.项目号"=w305:string, "Hopper car information.Hopper car code"=w304:string)
            n137 = Get Date/Time In Seconds() -> (seconds since 1Jan1904=w303:timestamp)
            n138 = Format Date/Time String(time format string (%c)="%y%m%d%H%M" ("时间格式字符串(%c)"), seconds (now)=w303) -> (date/time string=w301:string)  [unwired: 1 in]
            n139 = Concatenate Strings(w305, w304, w301) -> (w292:string)
            n140 = String Subset(string=w296, length (rest)=6 ("长度（剩余）")) -> (substring=w294:string)  [unwired: 1 in]
            n141 = call "Hopper car inf.vi"("write\\read（read)"=w297, "value"=w292, "key"=w296, "path in"=w299) -> ("path out"=w298:path)  [unwired: 6 in, 1 out]
            n142 = Build Array (concatenate)(w306, w305, w292) -> (w288:string[])
            n143 = Concatenate Strings(w294, "000") -> (w291:string)
            n144 = call "Hopper car inf.vi"("write\\read（read)"=w297, "value"=w292, "key"=w291, "path in"=w298) -> ()  [unwired: 6 in, 2 out]
            n145 = call "Creat XLS by Station.vi"("staiton"=Station."粗切工位", "data in"=w288) -> ("new file path (Not A Path if cancelled)"=w289:path)  [unwired: 4 in]
            n146 = Bundle By Name(cluster=w300, "database path"=w289) -> (w307:T3)
            n147 = Wait (ms)(milliseconds to wait=u32 100 ("等待时间（毫秒）")) -> ()  [unwired: 1 out]
          }
          frame "updata display" {
            n148 = Unbundle By Name(w314) -> ("rough cutting msic.粗切工位生产信息"=w316:refnum<vi>, "database path"=w315:path)
            n149 = call-poly <vilib>:"Read From Spreadsheet File.vi"("file path (dialog if empty)"=w315) -> ("all rows"=w313:string[][])  [unwired: 6 in, 4 out]
            n150 = Delete From Array(array=w313, length=1 ("长度"), index (row)=0 ("索引 (行)")) -> (array with subset deleted=w310:string[][])  [unwired: 1 in, 1 out]
            n151 = property class="Tbl (严格)"(reference=w316, "Value"=w310) -> ()  [unwired: 1 in, 2 out]
            n152 = Wait (ms)(milliseconds to wait=u32 100 ("等待时间（毫秒）")) -> ()  [unwired: 1 out]
          }
          frame "reset" {
            n153 = Unbundle By Name(w321) -> ("rough cutting msic.粗切条码"=w320:refnum<vi>)
            n154 = property class="Str"(reference=w320, "Value"="" ("值")) -> ()  [unwired: 1 in, 2 out]
            n155 = Bundle By Name(cluster=w321, "Number of scans"=u8 0, "pallet.produced number"=0, "BarCode"="", "Database"=string[] [], "Hopper car information"=T6 {"Hopper car code"="", "Hopper car No"="", "plate No"=""}) -> (w326:T3)
            n156 = Wait (ms)(milliseconds to wait=u32 100 ("等待时间（毫秒）")) -> ()  [unwired: 1 out]
          }
        }
        n157 = Unbundle By Name(w20) -> ("DsOut"=w19:T4[])
        n158 = property class="Str"(reference=w22, "Value"=w18) -> ()  [unwired: 1 in, 2 out]
        n159 = call-poly "Write Var To PLC.vi"("Tag IN"="PA10上位机当前状态", "String Var in"=w18, "Ds PLCTags IN"=w19) -> ()  [unwired: 1 in, 2 out]
        n160 = Wait (ms)(milliseconds to wait=u32 10 ("等待时间（毫秒）")) -> ()  [unwired: 1 out]
      }
    }
  }
